vi "CRYMessage Global.vi"() -> ()   [LabVIEW 2013]
panel:
  in  "Digital IO Port 2":u8 format="%x"
  in  "Digital IO Port 1":u8 format="%x"
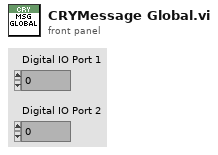
[diagram p1: front panel]
diagram:
